vi "FFT (SubVI).vi"(11 "Array in":dbl[](array[numeric])) -> (3 "Array out":dbl[](array[numeric]))   [LabVIEW 2011]
uses:
  <vilib>/Analysis/4window.llb/Hanning Window (DBL).vi
  <vilib>/Analysis/2dsp.llb/Real FFT.vi
  <vilib>/Analysis/NI_AALPro.lvlib
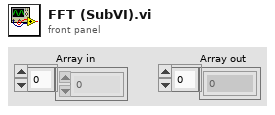
[diagram p1: front panel]
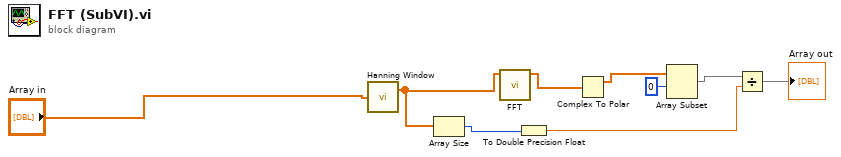
[diagram p0: block diagram]
diagram:
  n1 = call-poly <vilib>:"Hanning Window.vi"("X"="Array in") -> ("Windowed X"=w1:dbl[])  [unwired: 1 out]
  n2 = Array Size(array=w1) -> (size(s)=w4:i32)
  n3 = call-poly <vilib>:"FFT.vi"("X"=w1) -> ("FFT {X}"=w7:cdb[])  [unwired: 9 in, 1 out]
  n4 = To Double Precision Float(number=w4) -> (double precision float=w2:dbl)
  n5 = Complex To Polar(r * e^(i*theta)=w7) -> (r=w6:dbl[])  [unwired: 1 out]
  n6 = Array Subset(array=w6, index=0) -> (w3:dbl[])  [unwired: 1 in]
  n7 = Divide(x=w3, y=w2) -> (x/y=→"Array out":dbl[])
